vi "Select Device.vi"(11 "Devices":string[](array[string])) -> (2 "Cancelled?":bool, 3 "Device out":i32)   [LabVIEW 2020]
panel:
  in  "Cancel Button":bool
  in  "OK Button":bool
  in  "Device ring":i32(ring) items=["Andor", "Dummy", "IDS", "IMAQdx", "PCO Edge", "Scanner"]
  # "Hardware selection"
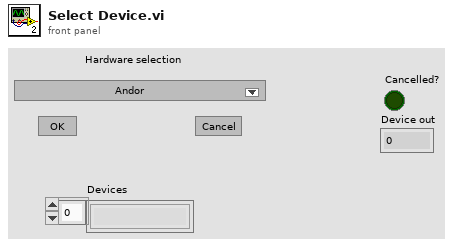
[diagram p1: front panel]
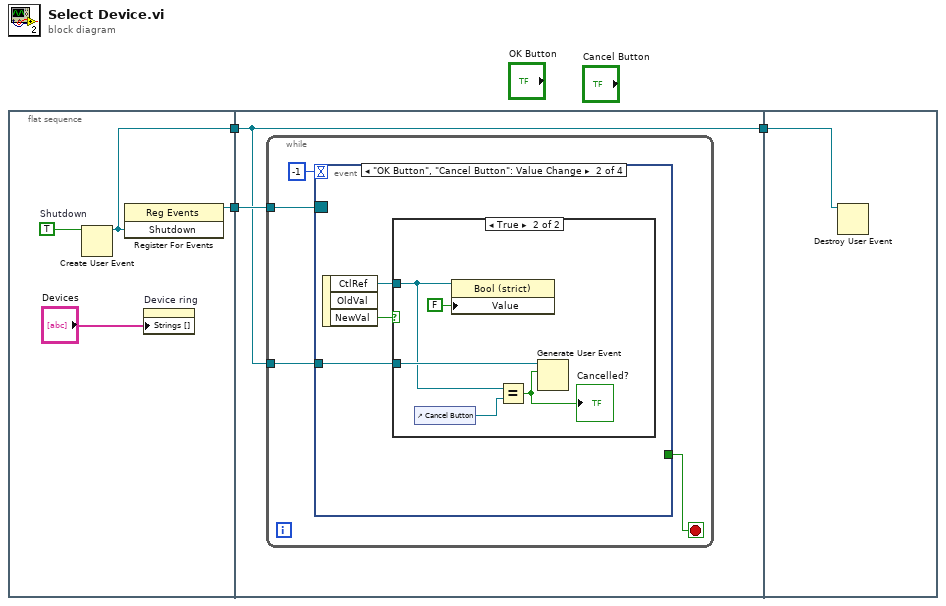
[diagram p0: block diagram]
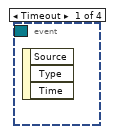
[diagram p2: hidden frame]
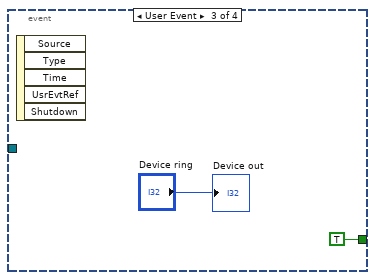
[diagram p4: hidden frame]
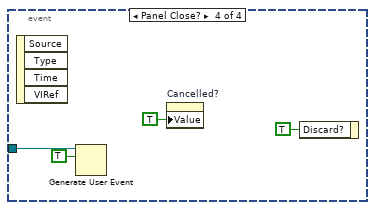
[diagram p5: hidden frame]
diagram:
  n1 = flat-sequence {
    tunnel: [w6] -> w3
    tunnel: [w4] -> w1
    tunnel: w3 -> [w9]
    tunnel: [w8] -> w2
    tunnel: w1 -> [w8]
    tunnel: w2 -> [w28]
    frame #0 {
      w5 = TRUE  # Shutdown
      n2 = Create User Event(user event datatype=w5) -> (user event=w4:refnum<user-event>)  [unwired: 1 in, 1 out]
      n3 = register-events(w4) -> (reference out=w6:refnum<event-registration>)  [unwired: 2 in, 1 out]
      n4 = property on="Device ring" class="Ring (strict)"("Strings []"="Devices") -> ()  [unwired: 2 in, 2 out]
    }
    frame #1 {
      n5 = while {
        tunnel: w9 -> [w11]
        tunnel: w8 -> [w10]
        stop <- w13 stop-if-true
        n6 = event shown="[1] \"OK Button\", \"Cancel Button\": Value Change" {
          selector: w11 -> [_ _ _ _]
          dyn-events: _ -> [_ _ _ _]
          timeout: -1 -> [_ _ _ _]
          tunnel: [_ _ TRUE _] -> w13
          tunnel: w10 -> [_ w14 _ w26]
          event Timeout {
            n7 = event-data() -> ()  [unwired: 1 in, 3 out]
          }
          event "OK Button", "Cancel Button": Value Change {
            n8 = event-data() -> ("CtlRef"=w16:refnum<vi>, "NewVal"=w15:bool)  [unwired: 1 in, 1 out]
            n9 = case shown="True" w15 {
              tunnel: w16 -> [_ w18]
              tunnel: w14 -> [_ w20]
              frame False {
              }
              frame True {
                n10 = control-ref of="Cancel Button"() -> (w19:refnum<vi>)
                n11 = property class="Bool (strict)"(reference=w18, "Value"=FALSE) -> ()  [unwired: 1 in, 2 out]
                n12 = Equal?(x=w18, y=w19) -> (x = y?=w17:bool)
                "Cancelled?" <- w17
                n13 = Generate User Event(user event=w20, event data cluster=w17) -> ()  [unwired: 2 in, 2 out]
              }
            }
          }
          event User Event {
            n14 = event-data() -> ()  [unwired: 1 in, 5 out]
            "Device out" <- "Device ring"
          }
          event Panel Close? {
            n15 = event-data() -> ()  [unwired: 1 in, 4 out]
            n16 = Generate User Event(user event=w26, event data cluster=TRUE ("event data")) -> ()  [unwired: 2 in, 2 out]
            n17 = property on="Cancelled?" class="Bool (strict)"("Value"=TRUE ("Cancelled?")) -> ()  [unwired: 2 in, 2 out]
            n18 = event-data("Discard?"=TRUE) -> ()  [unwired: 1 in, 1 out]
          }
        }
      }
    }
    frame #2 {
      n19 = Destroy User Event(user event=w28) -> ()  [unwired: 1 in, 1 out]
    }
  }
